vi "Read Drive Capacity.vi"(8 "error in (no error)":errorcluster, 11 "System Health Module in":refnum<class "System Health Module.lvclass">) -> (0 "error out":errorcluster, 3 "System Health Module out":refnum<class "System Health Module.lvclass">)   [LabVIEW 2020, in "Volatus.lvlib" / "System Health Module.lvclass"]
uses:
  System Health Module.lvclass
  System Health Module.lvclass/System Health Module.ctl
  System SAL/System SAL.lvclass
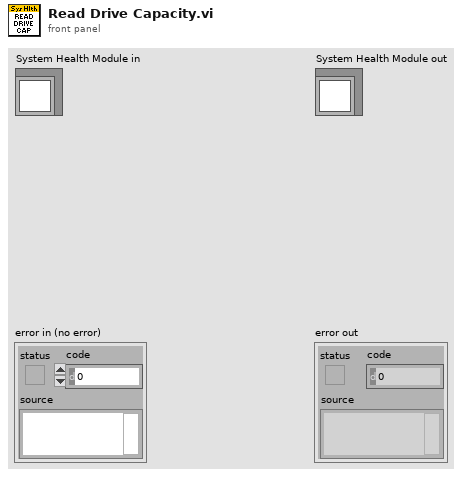
[diagram p1: front panel]
types:
  T1 = typedef "Volatus.lvlib/System Health Module.lvclass/Drive Info.ctl" = cluster{"Config":T2, "Capacity GB":dbl, "Used GB":dbl, "Next Warning":dbl, "Next Error":dbl}
  T2 = typedef "Volatus.lvlib/System Health Module.lvclass/Drive Config.ctl" = cluster{"Path":path, "Warning GB":dbl, "Error GB":dbl}
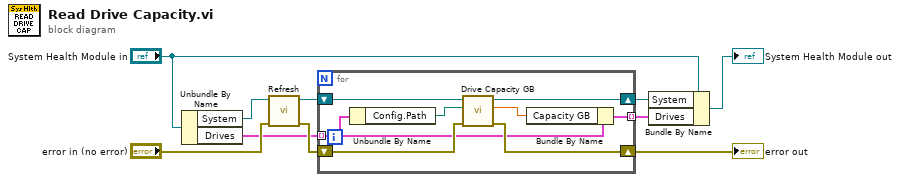
[diagram p0: block diagram]
diagram:
  n1 = Unbundle By Name("System Health Module in") -> ("System"=w7:refnum<class "System SAL.lvclass">, "Drives"=w6:T1[])
  n2 = call-dynamic "Refresh.vi"("error in (no error)"="error in (no error)", "System SAL in"=w7) -> ("error out"=w9:errorcluster, "System SAL out"=w1:refnum<class "System SAL.lvclass">)  [unwired: 8 in]
  n3 = for {
    shift-right: [w12] -> w4
    shift-left: w1 -> [w16]
    tunnel: w6 -> [w14] mode=indexing
    tunnel: [w11] -> w3 mode=indexing
    shift-right: [w17] -> w2
    shift-left: w9 -> [w18]
    n4 = Unbundle By Name(w14) -> ("Config.Path"=w15:path)
    n5 = call-dynamic "Drive Capacity GB.vi"("error in (no error)"=w18, "Path"=w15, "System SAL in"=w16) -> ("error out"=w17:errorcluster, "Capacity GB"=w13:dbl, "System SAL out"=w12:refnum<class "System SAL.lvclass">)  [unwired: 6 in]
    n6 = Bundle By Name(cluster=w14, "Capacity GB"=w13) -> (w11:T1)
  }
  "error out" <- w2
  n7 = Bundle By Name(cluster="System Health Module in", "System"=w4, "Drives"=w3) -> (→"System Health Module out":refnum<class "System Health Module.lvclass">)
